vi "Examples - AcquisitionTest_16Bit.vi"() -> ()   [LabVIEW 2015]
uses:
  xiLIB/xiCamLib/xiCam/PRM/IMG_FORMAT/IMG_DATA_FORMAT.ctl
  xiLIB/xiCamLib/xiCam/PRM/PRM/PRM_v2.ctl
panel:
  in  "Stop":bool
  out "Image":T1(plugin-control)
  # "Use this button instead of Abort Execution button"
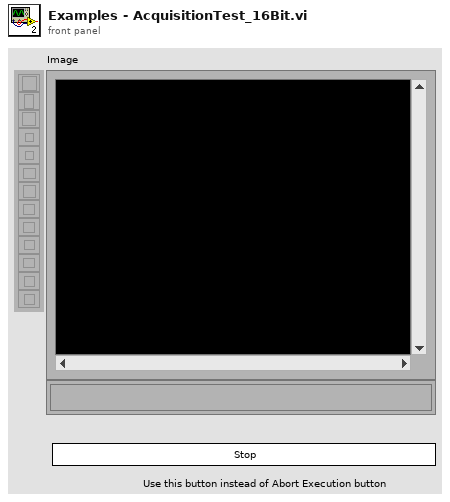
[diagram p1: front panel]
types:
  T1 = typedef "IMAQ Image.ctl" = refnum<image>
  T2 = typedef "PRM_v2.ctl" = enum16{"ACQ_BUFFER_SIZE", "ACQ_FRAME_BURST_COUNT", "ACQ_TIMING_MODE", "ACQ_TRANSPORT_BUFFER_SIZE", "AE_MAX_LIMIT", "AEAG", "AEAG_LEVEL", "API_VERSION", "AG_MAX_LIMIT", "APPLY_CMS", "AUTO_BANDWIDTH_CALCULATION", "AUTO_WB", "AVAILABLE_BANDWIDTH", "AVAILABLE_BANDWIDTH_MAX", "AVAILABLE_BANDWIDTH_MIN", "BPC", "BUFFER_POLICY", "BUFFERS_QUEUE_SIZE", "CC_MATRIX_00", "CC_MATRIX_01", "CC_MATRIX_02", "CC_MATRIX_03", "CC_MATRIX_10", "CC_MATRIX_11", "CC_MATRIX_12", "CC_MATRIX_13", "CC_MATRIX_20", "CC_MATRIX_21", "CC_MATRIX_22", "CC_MATRIX_23", "CC_MATRIX_30", "CC_MATRIX_31", "CC_MATRIX_32", "CC_MATRIX_33", "CHIP_TEMP", "CMS", "COLOR_FILTER_ARRAY", "COOLING", "DEBOUNCE_EN", "DEBOUNCE_POL", "DEBOUNCE_T0", "DEBOUNCE_T1", "DEBUG_LEVEL", "DEFAULT_CC_MATRIX", "DEVICE_INSTANCE_PATH", "DEVICE_MODEL_ID", "DEVICE_NAME", "DEVICE_SN", "DEVICE_TYPE", "DEVICE_USER_ID", "DOWNSAMPLING", "DOWNSAMPLING_MAX", "DOWNSAMPLING_MIN", "DOWNSAMPLING_TYPE", "DRV_VERSION", "EXP_PRIORITY", "EXPOSURE", "EXPOSURE_DIRECT_UPDATE", "EXPOSURE_MAX", "EXPOSURE_MIN", "FFS_FILE_NAME", "FPGA1_VERSION", "FRAMERATE", "FRAMERATE_MAX", "FRAMERATE_MIN", "FREE_FFS_SIZE", "GAIN", "GAIN_DIRECT_UPDATE", "GAIN_MAX", "GAIN_MIN", "GAMMAC", "GAMMAY", "GPI_LEVEL", "GPI_MODE", "GPI_SELECTOR", "GPI_SELECTOR_MAX", "GPI_SELECTOR_MIN", "GPO_MODE", "GPO_SELECTOR", "GPO_SELECTOR_MAX", "GPO_SELECTOR_MIN", "HDR", "HDR_T1", "HDR_T2", "HEIGHT", "HEIGHT_MAX", "HEIGHT_MIN", "HOUSE_TEMP", "IMAGE_DATA_FORMAT", "IMAGE_IS_COLOR", "INPUT_CMS_PROFILE", "IS_COOLED", "IS_DEVICE_EXIST", "KNEEPOINT1", "KNEEPOINT2", "LED_MODE", "LED_SELECTOR", "LED_SELECTOR_MAX", "LED_SELECTOR_MIN", "LIMIT_BANDWIDTH", "LIMIT_BANDWIDTH_MAX", "LIMIT_BANDWIDTH_MIN", "LUT_EN", "LUT_INDEX", "LUT_INDEX_MAX", "LUT_INDEX_MIN", "LUT_VALUE", "LUT_VALUE_MAX", "LUT_VALUE_MIN", "MANUAL_WB", "MCU1_VERSION", "MCU2_VERSION", "OFFSET_X", "OFFSET_X_MAX", "OFFSET_X_MIN", "OFFSET_Y", "OFFSET_Y_MAX", "OFFSET_Y_MIN", "OUTPUT_CMS_PROFILE", "OUTPUT_DATA_BIT_DEPTH", "OUTPUT_DATA_PACKING", "READ_FILE_FFS", "RECENT_FRAME", "SENSOR_DATA_BIT_DEPTH", "SENSOR_MODE", "SENSOR_TAPS", "SHARPNESS", "SHUTTER_TYPE", "TARGET_TEMP", "TRG_DELAY", "TRG_SELECTOR", "TRG_SOFTWARE", "TRG_SOURCE", "USED_FFS_SIZE", "WB_KB", "WB_KG", "WB_KR", "WIDTH", "WIDTH_MAX", "WIDTH_MIN", "WRITE_FILE_FFS", "ACQ_BUFFER_SIZE_UNIT", "ACQ_TRANSPORT_BUFFER_COMMIT", "AEAG_ROI_HEIGHT", "AEAG_ROI_OFFSET_X", "AEAG_ROU_OFFSET_Y", "AEAG_ROI_WIDTH", "API_CONTEXT_LIST", "BINNING_HORIZONTAL", "BINNING_SELECTOR", "BINNING_VERTICAL", "COLUMN_FPN_CORRECTION", "COUNTER_SELECTOR", "COUNTER_VALUE", "DECIMATION_HORIZONTAL", "DECIMATION_SELECTOR", "DECIMATION_VERTICAL", "DEVICE_ID", "DEVICE_LOCATION_PATH", "DEVICE_MANIFEST", "DEVICE_RESET", "DEVICE_SENS_SN", "EXPOSURE_BURST_COUNT", "FFS_ACCESS_KEY", "GAIN_SELECTOR", "HW_REVISION", "IMAGE_BLACK_LEVEL", "IMAGE_DATA_BIT_DEPTH", "IMAGE_DATA_FORMAT_RGB32_ALPHA", "IMAGE_PAYLOAD_SIZE", "LENS_APERTURE_VALUE", "LENS_FEATURE", "LENS_FEATURE_SELECTOR", "LENS_FOCAL_LENGTH", "LENS_FOCUS_DISTANCE", "LENS_FOCUS_MOVE", "LENS_FOCUS_MOVEMENT_VALUE", "LENS_MODE", "OUTPUT_DATA_PACKING_TYPE", "SENSOR_CLOCK_FREQ_HZ", "SENSOR_CLOCK_FREQ_INDEX", "SENSOR_FEATURE_SELECTOR", "SENSOR_FEATURE_VALUE", "SENSOR_OUTPUT_CHANNEL_COUNT", "TRANSPORT_PIXEL_FORMAT", "TS_RST_MODE", "TS_RST_SOURCE"}
  T3 = typedef "IMG_DATA_FORMAT.ctl" = enum16{"MONO8", "MONO16", "RGB24", "RGB32", "RGBPLANAR", "RAW8", "RAW16"}
  T4 = typedef "Image Type" = u32
  T5 = typedef "xiImageMng - Attributes.ctl" = cluster{"WIDTH":i32, "HEIGHT":i32, "IMG_FORMAT":T3}
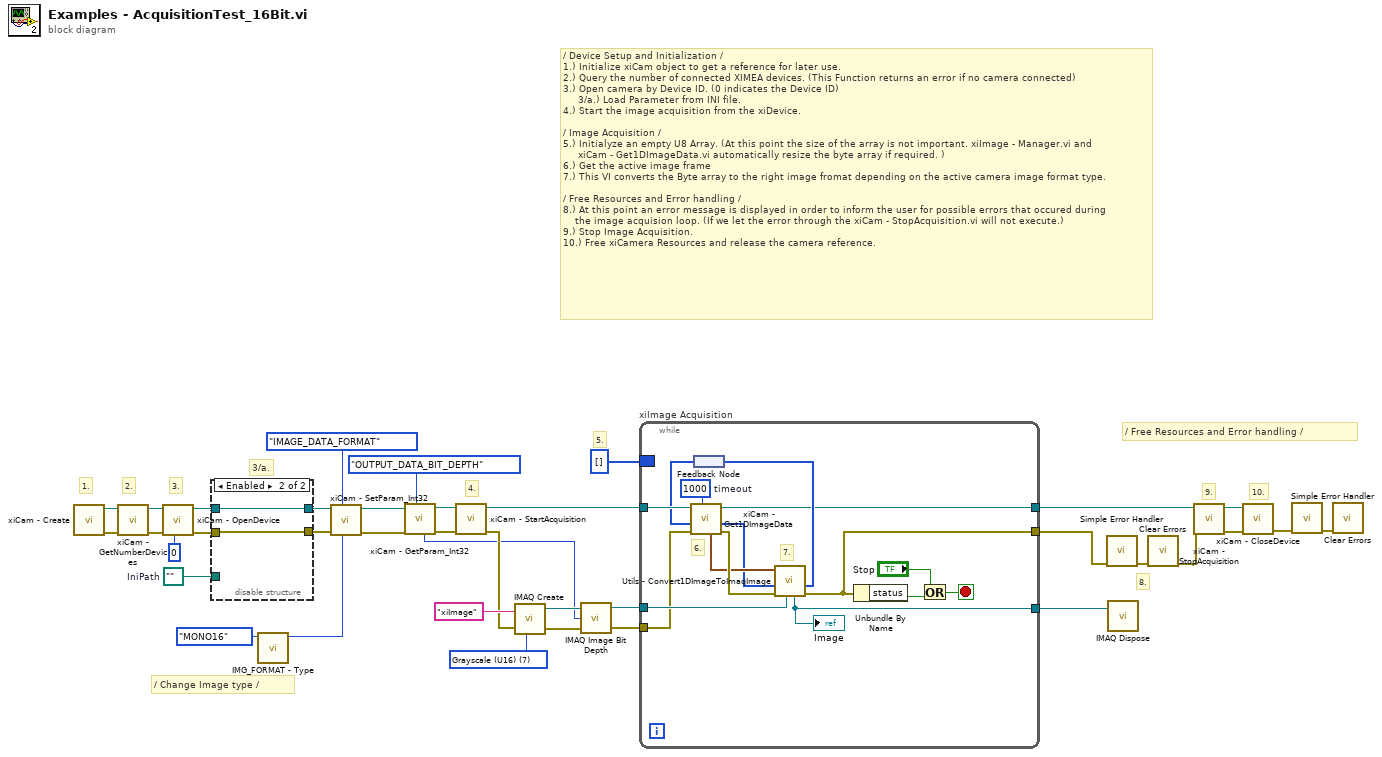
[diagram p0: block diagram]
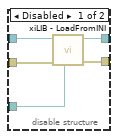
[diagram p2: hidden frame]
diagram:
  w16 = T4 7 items=["Grayscale (U8)", "Grayscale (I16)", "Grayscale (SGL)", "Complex (CSG)", "RGB (U32)", "HSL (U32)", "RGB (U64)", "Grayscale (U16)"] ("Image Type")
  w17 = path ""  # IniPath
  # "3/a."
  # "/ Free Resources and Error handling /"
  # "/ Change Image type /"
  # "9."
  # "10."
  # "8."
  # "5."
  # "/ Device Setup and Initialization /\n1.) Initialize xiCam object to get a reference for later use.\n2.) Query the number of connected XIMEA devices. (This Function returns an error if no camera connected)\n3.) Open camera by Device ID. (0 indicates the Device ID)\n     3/a.) Load Parameter from INI file. \n4.) Start the image acquisition from the xiDevice.\n\n/ Image Acquisition /\n5.) Initialyze an empty U8 Array. (At this point the size of the array is not important. xiImage - Manager.vi and\n     xiCam - Get1DImageData.vi automatically resize the byte array if required. )\n6.) Get the active image frame\n7.) This VI converts the Byte array to the right image fromat depending on the active camera image format type.\n\n/ Free Resources and Error handling /\n8.) At this point an error message is displayed in order to inform the user for possible errors that occured during\n    the image acquision loop. (If we let the error through the xiCam - StopAcquisition.vi will not execute.)\n9.) Stop Image Acquisition.\n10.) Free xiCamera Resources and release the camera reference."
  # "4."
  # "3."
  # "2."
  # "1."
  n1 = call "xiCam - Create.vi"() -> ("error out"=w36:errorcluster, "new xiCam"=w37:refnum<k24>)  [unwired: 10 in]
  n2 = call "xiCam - GetNumberDevices.vi"("error in (no error)"=w36, "xiCam In"=w37) -> ("error out"=w34:errorcluster, "xiCam Out"=w35:refnum<k24>)  [unwired: 7 in, 1 out]
  n3 = call "xiCam - OpenDevice.vi"("DevID"=0, "error in (no error)"=w34, "xiCam In"=w35) -> ("error out"=w18:errorcluster, "xiCam Out"=w19:refnum<k24>)  [unwired: 7 in]
  n4 = disable-structure shown="Enabled" {
    disable-tunnel: w19 -> [w42 w44]
    disable-tunnel: [w41 w44] -> w13
    disable-tunnel: [w40 w43] -> w12
    disable-tunnel: w18 -> [w39 w43]
    disable-tunnel: w17 -> [w38 _]
    frame Disabled {
      n5 = call "xiLIB - LoadFromINI.vi"("IniPath"=w38, "Error In"=w39, "xiCam In"=w42) -> ("Error Out"=w40:errorcluster, "xiCam Out"=w41:refnum<k24>)  [unwired: 7 in]
    }
    frame Enabled {
    }
  }
  n6 = call "IMG_FORMAT - Type.vi"("IMG_FORMAT"=IMG_DATA_FORMAT."MONO16") -> ("IMG_FORMAT_VALUE"=w11:i32)  [unwired: 9 in, 1 out]
  n7 = call "xiCam - SetParam_Int32.vi"("Int32_Value"=w11, "PRM"=PRM_v2."IMAGE_DATA_FORMAT", "error in (no error)"=w12, "xiCam In"=w13) -> ("error out"=w9:errorcluster, "xiCam Out"=w10:refnum<k24>)  [unwired: 6 in]
  n8 = call "xiCam - GetParam_Int32.vi"("PRM"=PRM_v2."OUTPUT_DATA_BIT_DEPTH", "error in (no error)"=w9, "xiCam In"=w10) -> ("error out"=w8:errorcluster, "xiCam Out"=w7:refnum<k24>, "Int32_Value"=w1:i32)  [unwired: 6 in]
  n9 = call "xiCam - StartAcquisition.vi"("error in (no error)"=w8, "xiCam In"=w7) -> ("error out"=w21:errorcluster, "xiCam Out"=w32:refnum<k24>)  [unwired: 8 in]
  n10 = call "IMAQ Create"("Image Name"="xiImage", "Image Type"=w16, "error in (no error)"=w21) -> ("New Image"=w5:T1, "error out"=w3:errorcluster)  [unwired: 2 in]
  n11 = call "IMAQ Image Bit Depth"("Image"=w5, "Bit Depth (0)"=w1, "error in (no error)"=w3) -> ("Image Out"=w4:T1, "error out"=w2:errorcluster)  [unwired: 10 in, 1 out]
  n12 = while "xiImage Acquisition" {
    tunnel: w32 -> [w59]
    border: u8[] [] ("1DImageData Out") -> [_]
    tunnel: [w49] -> w29
    tunnel: [w48] -> w30
    tunnel: w4 -> [w47]
    tunnel: w2 -> [w46]
    tunnel: [w45] -> w20
    stop <- w50 stop-if-true
    w57 = 1000  # timeout
    # "7."
    # "6."
    n13 = feedback #1() -> (w58:u8[])
    n14 = call "xiCam - Get1DImageData.vi"("timeout"=w57, "error in (no error)"=w46, "1DImageData In"=w58, "xiCam In"=w59) -> ("error out"=w56:errorcluster, "1DImageData Out"=w54:u8[], "xiCam Out"=w48:refnum<k24>, "Image Properites"=w55:T5)  [unwired: 4 in]
    n15 = call "Utils - Convert1DImageToImaqImage.vi"("Image In"=w47, "error in (no error)"=w56, "1DImageData In"=w54, "Image Properties In"=w55) -> ("error out"=w49:errorcluster, "1DImageData Out"=w53:u8[], "Image Out"=w45:T1)  [unwired: 5 in]
    "Image" <- w45
    n16 = feedback-in #1(w53) -> ()
    n17 = Unbundle By Name(w49) -> ("status"=w52:bool)
    n18 = Or(x="Stop", y=w52) -> (x .or. y?=w50:bool)
  }
  n19 = call <vilib>:"Simple Error Handler.vi"("error in (no error)"=w29) -> ("error out"=w28:errorcluster)  [unwired: 4 in, 4 out]
  n20 = call "IMAQ Dispose"("Image"=w20) -> ()  [unwired: 5 in, 1 out]
  n21 = call <vilib>:"Clear Errors.vi"("error in (no error)"=w28) -> ("error out"=w27:errorcluster)  [unwired: 5 in, 1 out]
  n22 = call "xiCam - StopAcquisition.vi"("error in (no error)"=w27, "xiCam In"=w30) -> ("error out"=w25:errorcluster, "xiCam Out"=w26:refnum<k24>)  [unwired: 8 in]
  n23 = call "xiCam - CloseDevice.vi"("error in (no error)"=w25, "xiCam In"=w26) -> ("error out"=w23:errorcluster)  [unwired: 9 in]
  n24 = call <vilib>:"Simple Error Handler.vi"("error in (no error)"=w23) -> ("error out"=w24:errorcluster)  [unwired: 4 in, 4 out]
  n25 = call <vilib>:"Clear Errors.vi"("error in (no error)"=w24) -> ()  [unwired: 5 in, 2 out]
